vi "Channel_name_checker.vi"(2 "Email On Error?":bool, 3 "Channel names":string[](array[string])) -> (0 "No of Errors":i32, 1 "Channel names Out":string[](array[string]))   [LabVIEW 2010]
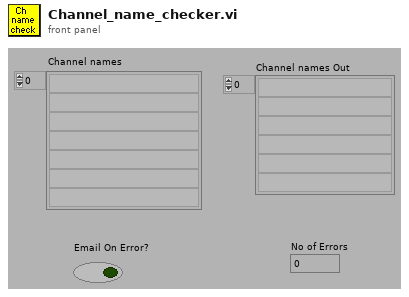
[diagram p1: front panel]
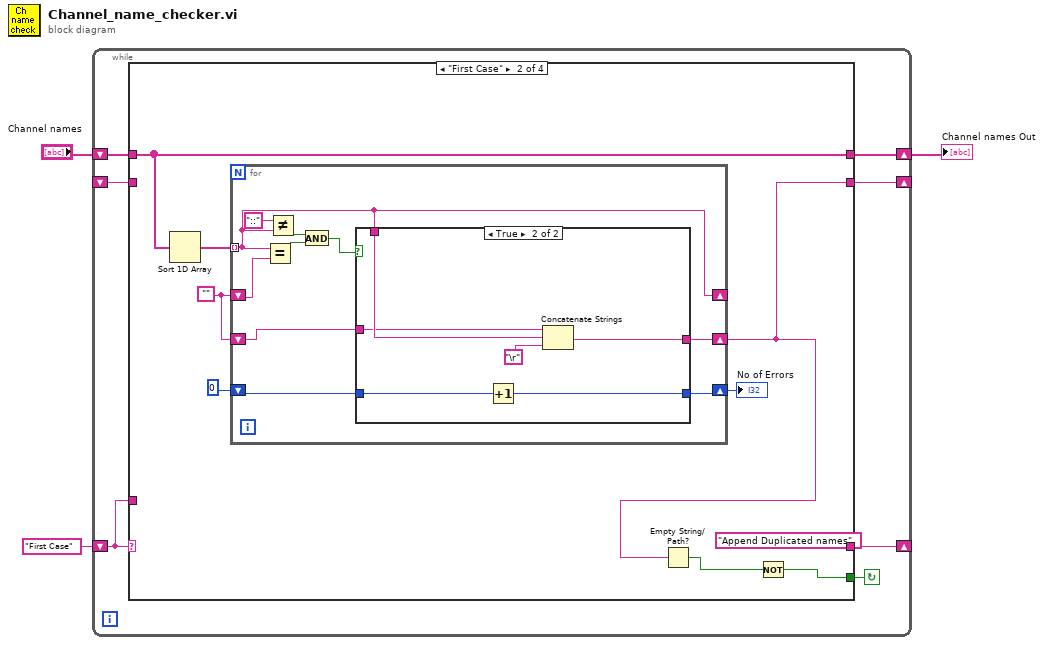
[diagram p0: block diagram]
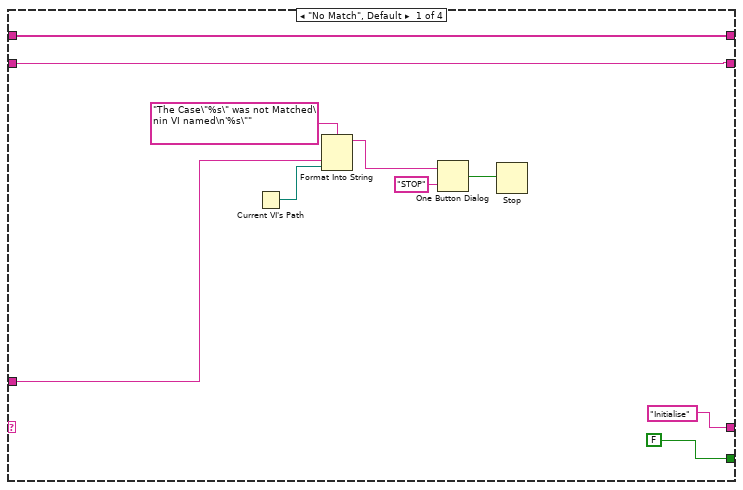
[diagram p2: hidden frame]
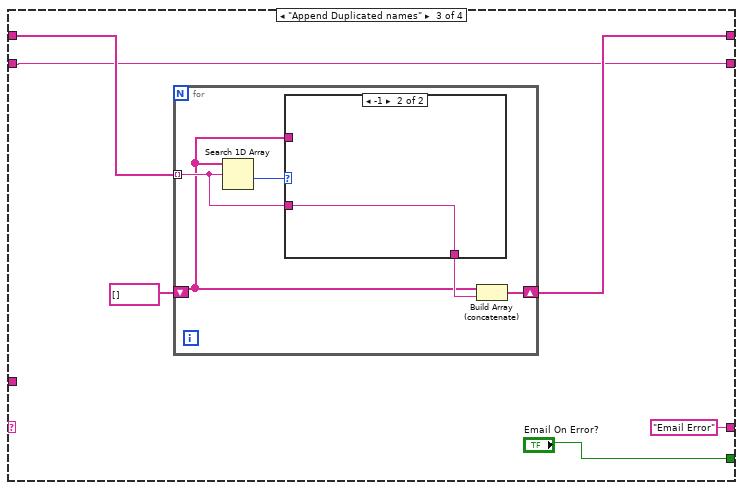
[diagram p4: hidden frame]
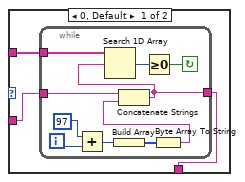
[diagram p5: hidden frame]
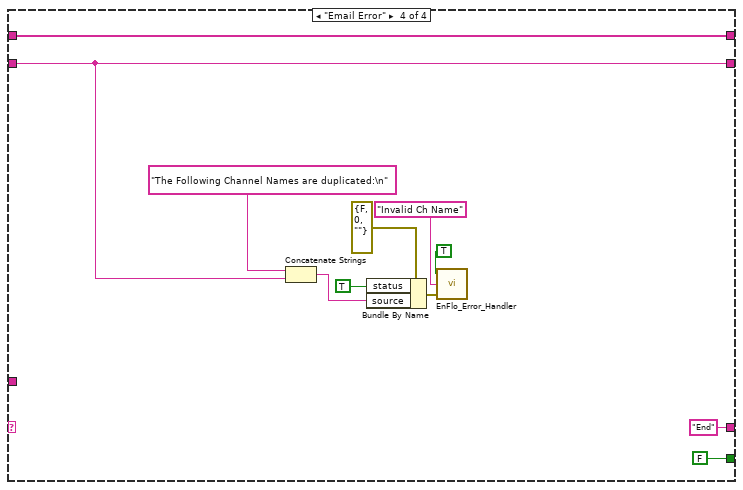
[diagram p6: hidden frame]
diagram:
  n1 = while {
    shift-left: "First Case" -> [w8]
    shift-right: [w9] -> _
    shift-right: [w5] -> w1
    shift-left: "Channel names" -> [w7]
    shift-right: [w6] -> _
    shift-left: _ -> [w4]
    stop <- w10 continue-if-true
    n2 = case shown="\"First Case\"" w8 {
      tunnel: [FALSE w21 "Email On Error?" FALSE ("Email On Error?")] -> w10
      tunnel: ["Initialise" "Append Duplicated names" "Email Error" "End"] -> w9
      tunnel: w8 -> [w15 _ _ _]
      tunnel: w7 -> [w12 w24 w52 w75]
      tunnel: [w11 w23 w50 w76] -> w6
      tunnel: [w12 w24 w51 w75] -> w5
      tunnel: w4 -> [w11 _ w50 w76]
      frame "No Match", Default {
        n3 = Current VI's Path() -> (path=w14:path)
        n4 = Format Into String(format string="The Case\"%s\" was not Matched\nin VI named\n'%s\"" ("Format String"), w15, w14) -> (resulting string=w18:string)  [unwired: 2 in, 1 out]
        n5 = One Button Dialog(message=w18, button name ("OK")="STOP") -> (true=w16:bool)
        n6 = Stop(stop? (T)=w16) -> ()
      }
      frame "First Case" {
        w28 = ""
        n7 = Sort 1D Array(array=w24) -> (sorted array=w25:string[])
        n8 = for {
          shift-right: [w38] -> _
          shift-left: w28 -> [w39]
          tunnel: w25 -> [w38] mode=indexing
          shift-right: [w32] -> w27
          shift-left: 0 -> [w33]
          shift-right: [w30] -> w23
          shift-left: w28 -> [w31]
          n9 = Equal?(x=w38, y=w39) -> (x = y?=w35:bool)
          n10 = Not Equal?(x="::", y=w38) -> (x != y?=w36:bool)
          n11 = And(x=w36, y=w35) -> (x .and. y?=w34:bool)
          n12 = case shown="True" w34 {
            tunnel: w38 -> [_ w45]
            tunnel: w33 -> [w41 w47]
            tunnel: [w41 w46] -> w32
            tunnel: w31 -> [w40 w44]
            tunnel: [w40 w43] -> w30
            frame False {
            }
            frame True {
              n13 = Increment(x=w47) -> (x+1=w46:i32)
              n14 = Concatenate Strings(w44, w45, "\r") -> (w43:string)
            }
          }
        }
        "No of Errors" <- w27
        n15 = Empty String/Path?(string/path=w23) -> (empty?=w22:bool)
        n16 = Not(x=w22) -> (.not. x?=w21:bool)
      }
      frame "Append Duplicated names" {
        n17 = for {
          shift-right: [w56] -> w51
          shift-left: string[] [] -> [w54]
          tunnel: w52 -> [w55] mode=indexing
          n18 = Search 1D Array(1D array=w54, element=w55) -> (index of element=w58:i32)  [unwired: 1 out]
          n19 = case shown="-1" w58 {
            tunnel: [w59 w72] -> w57
            tunnel: w55 -> [w61 w72]
            tunnel: w54 -> [w60 _]
            frame 0, Default {
              n20 = while {
                tunnel: [w62] -> w59
                tunnel: w60 -> [w65]
                tunnel: w61 -> [w66]
                i -> [w67]
                stop <- w63 continue-if-true
                n21 = Add(x=97, y=w67) -> (x+y=w70:i32)
                n22 = Build Array(w70) -> (w71:i32[])
                n23 = Byte Array To String(unsigned byte array=w71) -> (string=w68:string)
                n24 = Concatenate Strings(w66, w68) -> (w62:string)
                n25 = Search 1D Array(1D array=w65, element=w62) -> (index of element=w64:i32)  [unwired: 1 out]
                n26 = Greater Or Equal To 0?(x=w64) -> (x >= 0?=w63:bool)
              }
            }
            frame -1 {
            }
          }
          n27 = Build Array (concatenate)(w54, w57) -> (w56:string[])
        }
      }
      frame "Email Error" {
        n28 = Concatenate Strings("The Following Channel Names are duplicated:\n", w76) -> (w81:string)
        n29 = Bundle By Name(cluster=errorcluster {"status"=FALSE, "code"=0, "source"=""} ("error in (no error)"), "status"=TRUE ("Bundle Element"), "source"=w81) -> (w79:errorcluster)
        n30 = call "EnFlo_Error_Handler.vi"("error in (no error)"=w79, "Error Type"="Invalid Ch Name", "Dialog Box (T)"=TRUE ("Dialog Box")) -> ()  [unwired: 3 out]
      }
    }
  }
  "Channel names Out" <- w1
